vi "confirmINIsettings.vi"() -> ()   [LabVIEW 2012]
doc: "SciScan 1.2 160622"
uses:
  <vilib>/Utility/config.llb/Read Key (String).vi
  GFG/GFGpathGet.vi
  <vilib>/Utility/config.llb/Write Key (Boolean).vi
  <vilib>/Utility/config.llb/Read Key (Boolean).vi
  <vilib>/Utility/config.llb/Write Key (String).vi
  GFG/GFG library.lvlib
  <vilib>/Utility/config.llb/NI_LVConfig.lvlib
panel:
  in  "Fresh config or upgrade?":enum32{"Fresh", "Upgrade"}(radio) caption="1) Start a complete new configuration?"
  in  "PhotoStim Shutter Port":tag="PXI1Slot4/port0/line0" caption="4) Specify the shutter port for the photo stimulation light path"
  in  "DAQ Package":T1(ring) caption="2) Select a DAQ package"
  out "Written files":path[](array[path])
  in  "Load INI variables":bool caption="5) Select optional modules and confirm hardware"
  out "Reso settings complete?":bool
  out "Galvo settings complete?":bool
  out "Loaded scanner configuration":string
  in  "Select modules and confirm hardware":bool caption="6) Select modules and confirm hardware"
  out "Previous INI file settings":path caption="Previous SciScan root path (optional)"
  out "INI to write at....":path
  in  "EXIT":bool
  in  "Switch (Linkbone) Serial Port":refnum<visa-resource-name>=" " caption="3) Specify the detector switch COM port (Linkbone)"
  # "R - Resonant scan mirror   G - Galvo scan mirror"
  # "SciScan Configuration Tool"
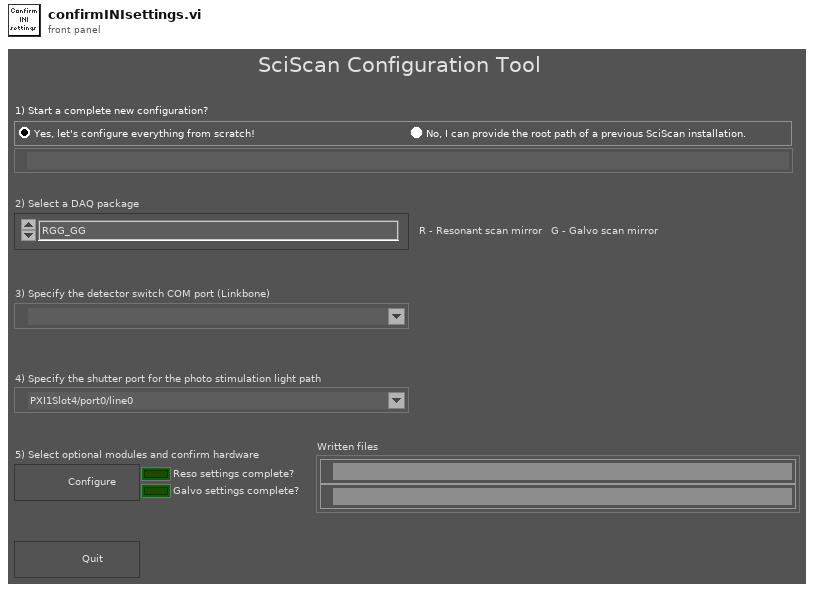
[diagram p1: front panel]
types:
  T1 = enum16{"RGG_GG", "RG_GG", "GG_GG", "RGG", "RG (standalone)", "GG (standalone)"}
  T2 = enum32{"invalid OS target", "Mac OS", "Windows 3.1", "Windows 95/NT", "Solaris 1", "Solaris 2", "HP-UX", "PowerMAX", "Linux", "Irix", "Rhapsody", "BeOS", "AIX", "OSF1", "VxWorks", "PharLap", "Carbon", "RTX", "Windows x64", "Linux x64"}
  T3 = enum8{"Enabled", "Disabled", "Disabled and Grayed Out"}
  T4 = typedef "NI_LVConfig.lvlib/Config Data RefNum.ctl" = refnum<k1>
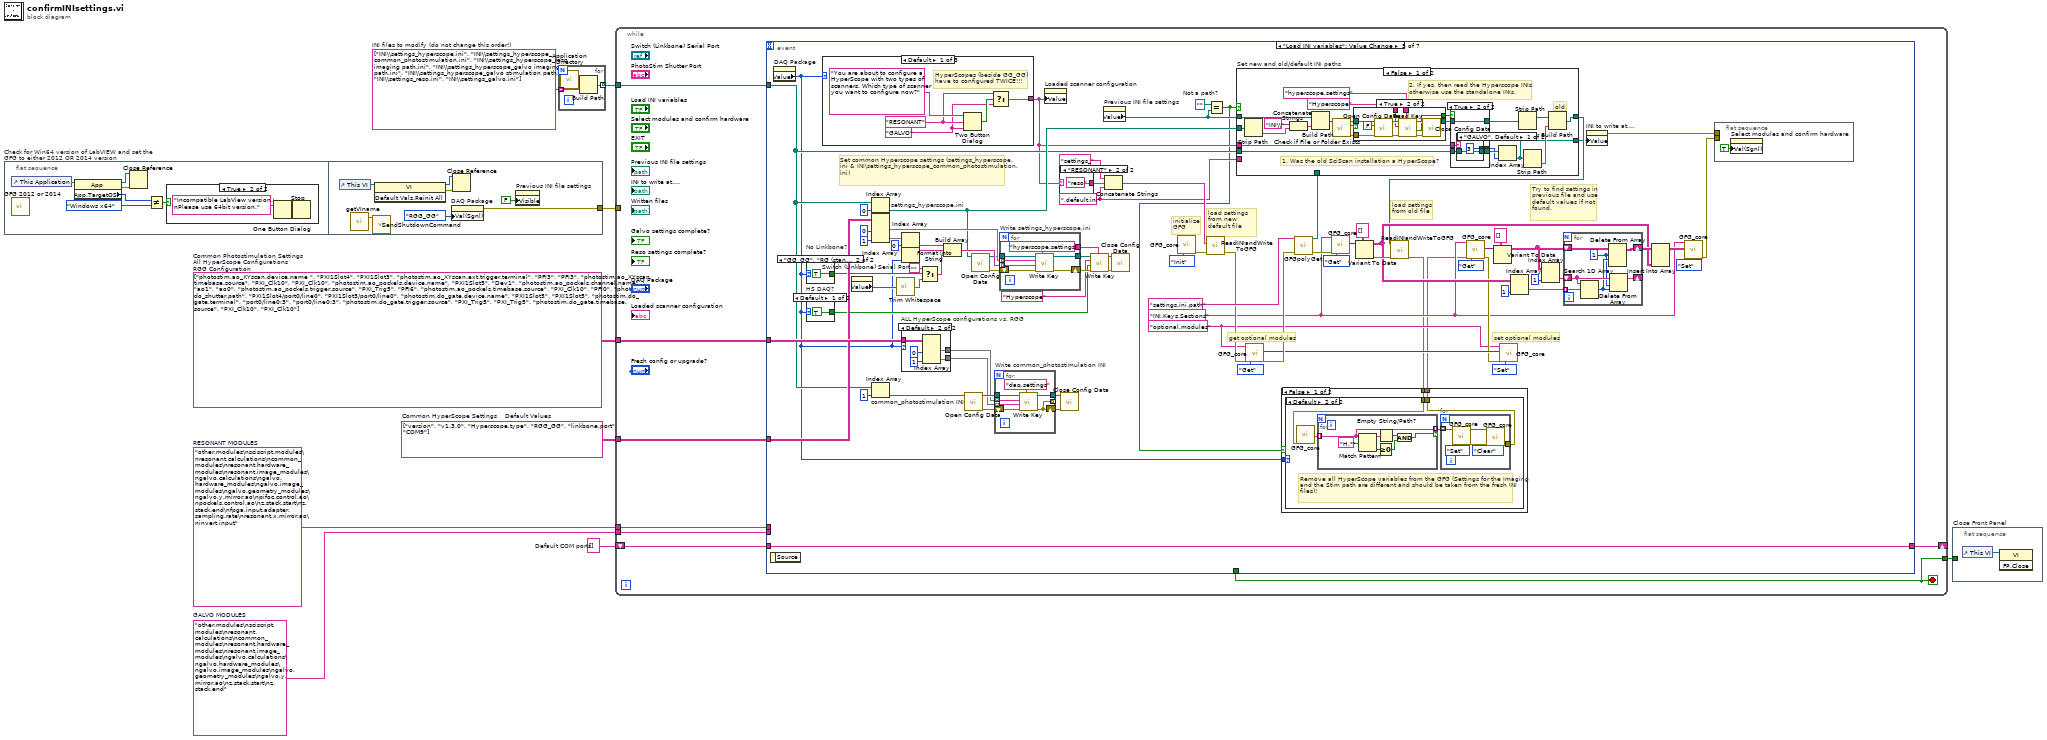
[diagram p0: block diagram]
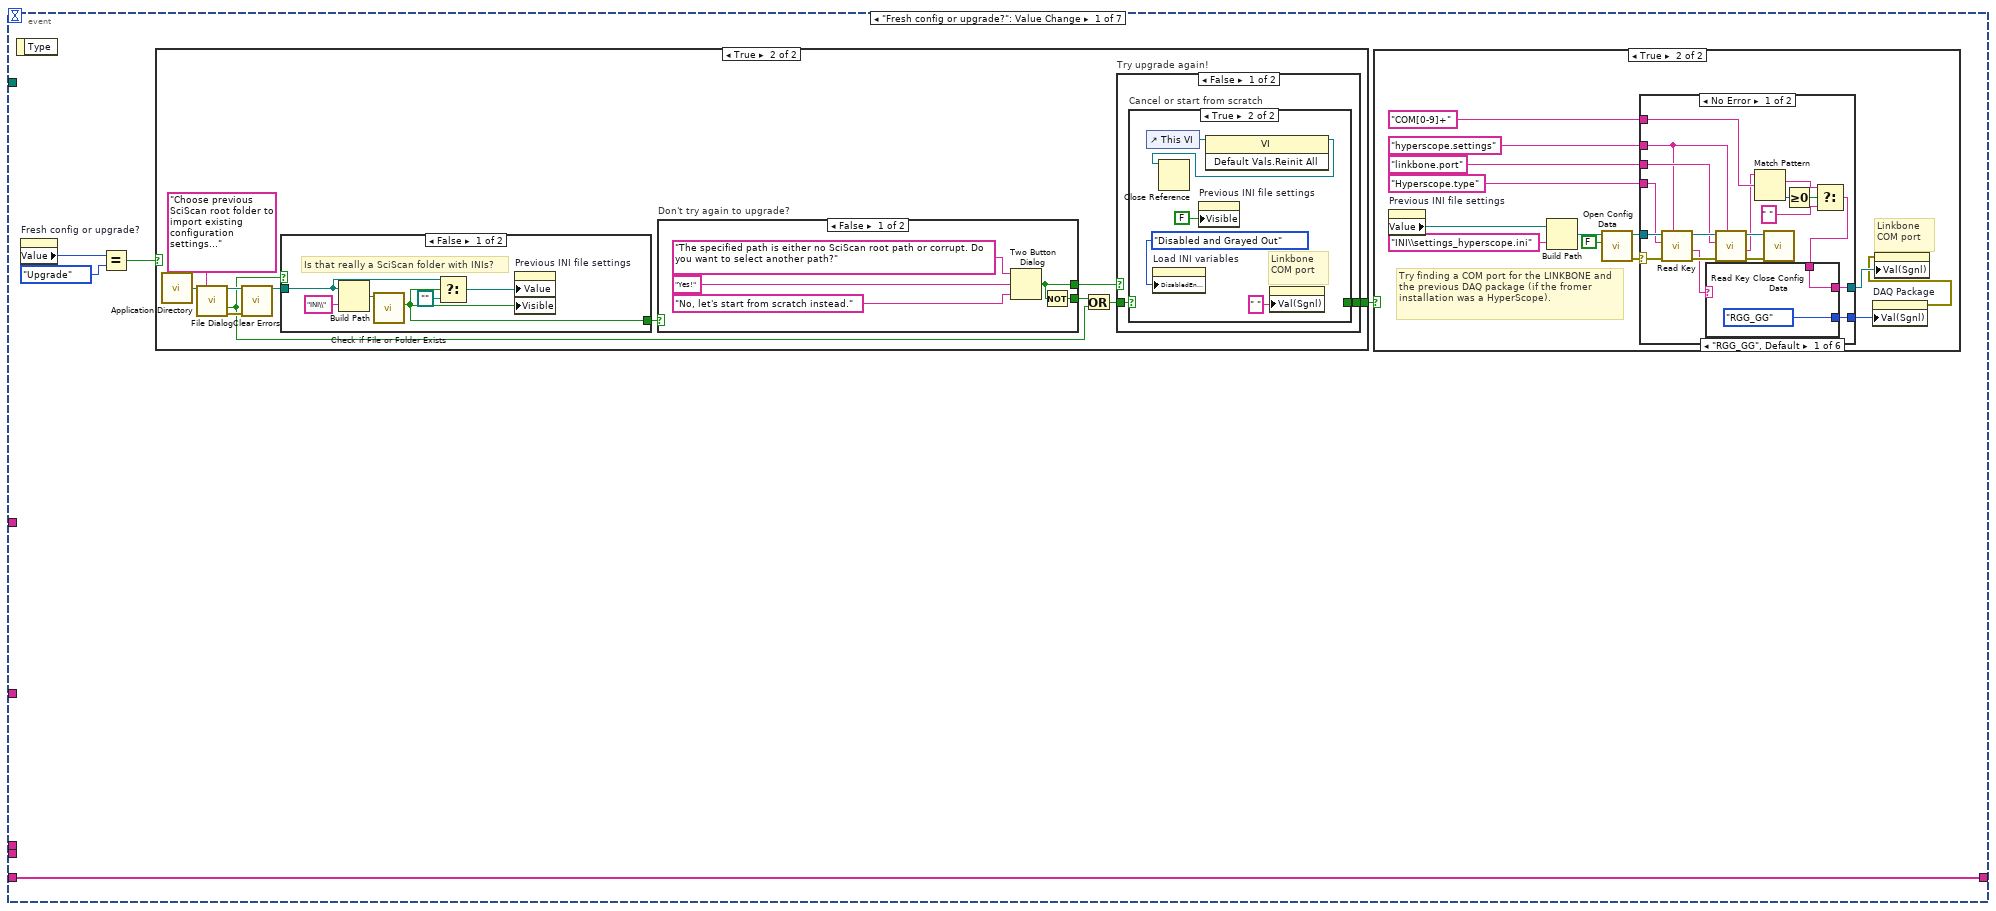
[diagram p3: hidden frame]
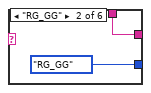
[diagram p5: hidden frame]
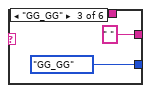
[diagram p6: hidden frame]
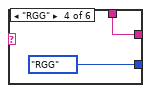
[diagram p7: hidden frame]
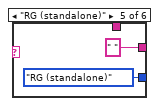
[diagram p8: hidden frame]
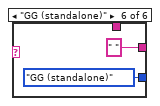
[diagram p9: hidden frame]
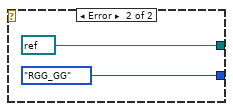
[diagram p10: hidden frame]
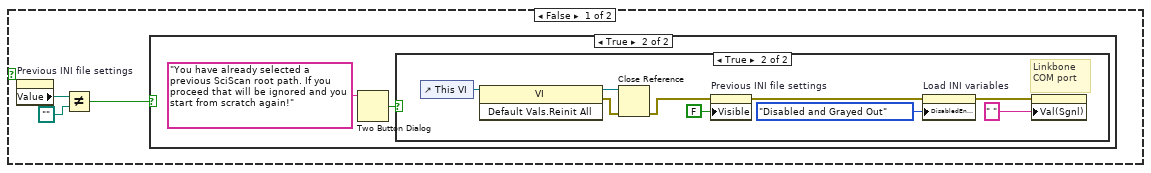
[diagram p11: hidden frame]
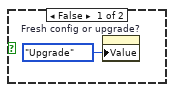
[diagram p13: hidden frame]
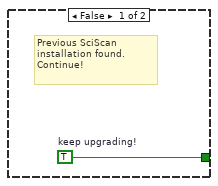
[diagram p15: hidden frame]
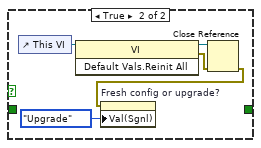
[diagram p16: hidden frame]
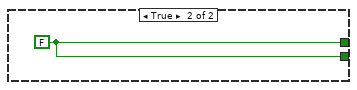
[diagram p17: hidden frame]
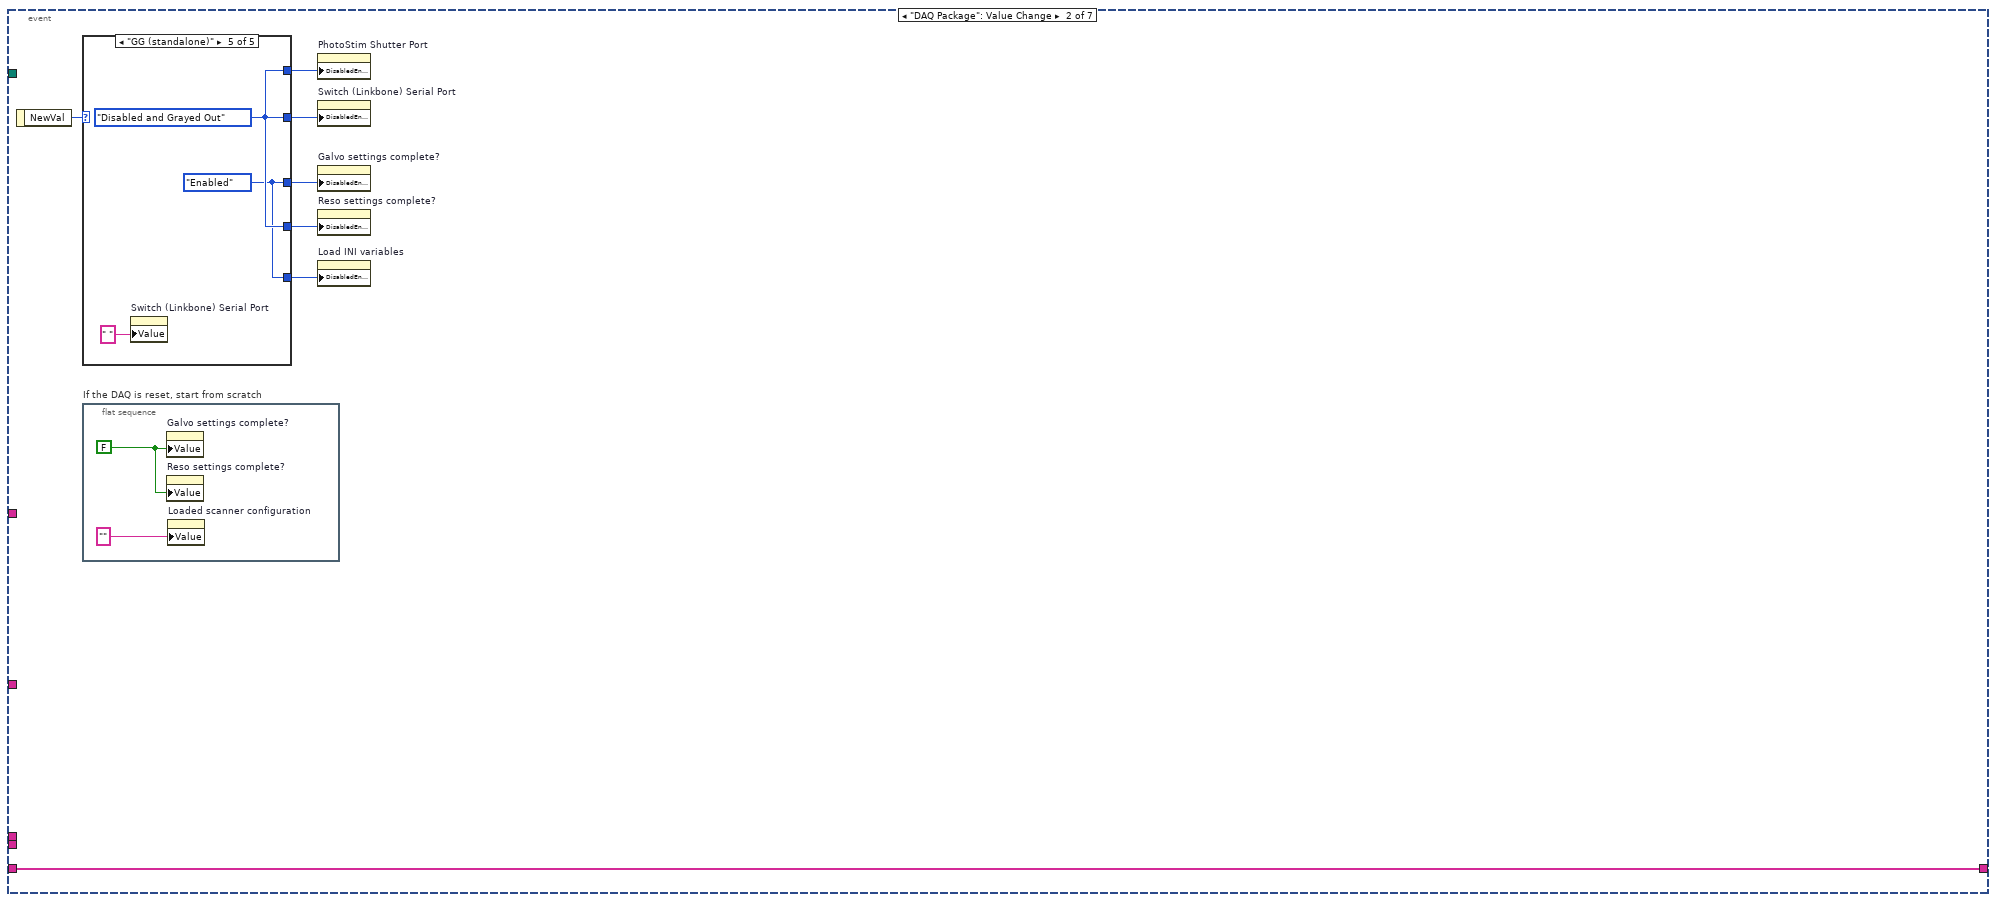
[diagram p18: hidden frame]
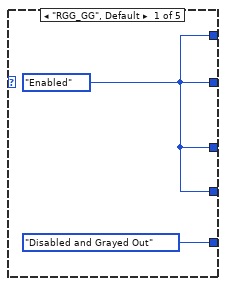
[diagram p19: hidden frame]
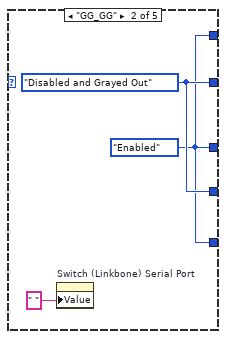
[diagram p20: hidden frame]
diagram:
  w1 = string[] []  # Default COM ports
  w2 = "other.modules\nsciscript.modules\nresonant.calculations\ncommon_modules\nresonant.hardware_modules\nresonant.image_modules\ngalvo.calculations\ngalvo.hardware_modules\ngalvo.image_modules\ngalvo.geometry_modules\ngalvo.y.mirror.ao\npifoc.control.ao\npockels.control.ao\nz.stack.start\nz.stack.end\nfpga.input.adapter.sampling.rate\nresonant.x.mirror.ao\ninvert.input"  # RESONANT MODULES
  w3 = "other.modules\nsciscript.modules\nresonant.calculations\ncommon_modules\nresonant.hardware_modules\nresonant.image_modules\ngalvo.calculations\ngalvo.hardware_modules\ngalvo.image_modules\ngalvo.geometry_modules\ngalvo.y.mirror.ao\nz.stack.start\nz.stack.end"  # GALVO MODULES
  w4 = string[][] [["version", "v1.3.0"], ["Hyperscope.type", "RGG_GG"], ["linkbone.port", "COM9"]]  # Common HyperScope Settings    Default Values
  w7 = string[] ["INI\\settings_hyperscope.ini", "INI\\settings_hyperscope_common_photostimulation.ini", "INI\\settings_hyperscope_reso imaging path.ini", "INI\\settings_hyperscope_galvo imaging path.ini", "INI\\settings_hyperscope_galvo stimulation path.ini", "INI\\settings_reso.ini", "INI\\settings_galvo.ini"]  # INI files to modify (do not change this order!)
  w5 = string[][] [["photostim.ao_XYscan.device.name ", "PXI1Slot4", "PXI1Slot3"], ["photostim.ao_XYscan.ext.trigger.terminal", "PFI3", "PFI3"], ["photostim.ao_XYscan.timebase.source", "PXI_Clk10", "PXI_Clk10"], ["photostim.ao_pockels.device.name", "PXI1Slot5", "Dev1"], ["photostim.ao_pockels.channel.name", "ao1", "ao0"], ["photostim.ao_pockels.trigger.source", "PXI_Trig5", "PFI6"], ["photostim.ao_pockels.timebase.source", "PXI_Clk10", "PFI0"], ["photostim.do_shutter.path", "PXI1Slot4/port0/line0", "PXI1Slot3/port0/line0"], ["photostim.do_gate.device.name", "PXI1Slot5", "PXI1Slot5"], ["photostim.do_gate.terminal", "port0/line0:3", "port0/line0:3"], ["photostim.do_gate.trigger.source", "PXI_Trig5", "PXI_Trig5"], ["photostim.do_gate.timebase.source", "PXI_Clk10", "PXI_Clk10"]]  # Common Photostimulation Settings                 All HyperScope Configurations                       RGG Configuration
  n1 = flat-sequence "Check for Win64 version of LabVIEW and set the GFG to either 2012 OR 2014 version" {
    tunnel: [w20] -> w8
    frame #0 {
      n2 = control-ref of="This Application"() -> (w10:refnum<vi>)
      n3 = call "GFG 2012 or 2014.vi"() -> ()  [unwired: 12 in]
      n4 = property class="App"(reference=w10) -> (reference out=w14:refnum<vi>, error out=w15:errorcluster, "App.TargetOS"=w11:T2)  [unwired: 1 in]
      n5 = Close Reference(reference=w14, error in (no error)=w15) -> ()  [unwired: 1 out]
      n6 = Not Equal?(x=w11, y=T2."Windows x64" ("Application:Target:Operating System")) -> (x != y?=w13:bool)
      n7 = case shown="True" w13 {
        frame False {
        }
        frame True {
          n8 = One Button Dialog(message="Incompatible LabView version.\nPlease use 64bit version." ("source")) -> (true=w16:bool)  [unwired: 1 in]
          n9 = Stop(stop? (T)=w16) -> ()
        }
      }
    }
    frame #1 {
      n10 = control-ref of="This VI"() -> (w22:refnum<vi>)
      n11 = call "getVIname.vi"() -> ("VI name"=w24:string)  [unwired: 19 in]
      n12 = call "SendShutdownCommand.vi"("Source VI"=w24) -> ()  [unwired: 11 in]
      n13 = invoke class="VI" method="Default Vals.Reinit All"(reference=w22) -> (reference out=w19:refnum<vi>, error out=w18:errorcluster)  [unwired: 2 in, 1 out]
      n14 = property on="DAQ Package" class="Enum (strict)"("Val(Sgnl)"=enum16{"RGG_GG", "RG_GG", "GG_GG", "RGG"}."RGG_GG" ("DAQ Package")) -> (error out=w20:errorcluster)  [unwired: 2 in, 1 out]
      n15 = Close Reference(reference=w19, error in (no error)=w18) -> ()  [unwired: 1 out]
      n16 = property on="Previous INI file settings" class="Path"("Visible"=FALSE) -> ()  [unwired: 2 in, 2 out]
    }
  }
  n17 = for {
    tunnel: w7 -> [w26] mode=indexing
    tunnel: [w25] -> w6 mode=indexing
    n18 = call <vilib>:"Application Directory.vi"() -> ("Application Directory"=w27:path)
    n19 = Build Path(base path=w27, name or relative path=w26) -> (appended path=w25:path)
  }
  n20 = while {
    tunnel: [w35] -> w9
    tunnel: w5 -> [w34]
    tunnel: w8 -> [_]
    tunnel: w6 -> [w33]
    tunnel: w4 -> [w32]
    tunnel: w3 -> [w31]
    tunnel: w2 -> [w30]
    shift-right: [w28] -> _
    shift-left: w1 -> [w29]
    stop <- w35 stop-if-true
    n21 = event shown="[4] \"Load INI variables\": Value Change" {
      selector: _ -> [_ _ _ _ _ _ _]
      dyn-events: _ -> [_ _ _ _ _ _ _]
      timeout: _ -> [_ _ _ _ _ _ _]
      tunnel: [_ _ _ _ _ _ w528] -> w35
      tunnel: w34 -> [_ _ _ _ w251 _ _]
      tunnel: w33 -> [_ _ _ _ w186 w393 _]
      tunnel: w32 -> [_ _ _ _ w250 _ _]
      tunnel: w31 -> [_ _ _ _ _ w396 _]
      tunnel: w30 -> [_ _ _ _ _ w395 _]
      tunnel: w29 -> [w40 w139 w166 w169 w248 w381 w527]
      tunnel: [w40 w139 w166 w169 w248 w380 w527] -> w28
      event "Fresh config or upgrade?": Value Change {
        n22 = event-data() -> ()  [unwired: 1 in, 1 out]
        n23 = property on="Fresh config or upgrade?" class="RadioBtnsControl (strict)"() -> ("Value"=w39:enum32{"Fresh", "Upgrade"})  [unwired: 2 in, 2 out]
        n24 = Equal?(x=w39, y=enum32{"Fresh", "Upgrade"}."Upgrade") -> (x = y?=w37:bool)
        n25 = case shown="True" w37 {
          tunnel: [_ w102] -> w36
          frame False {
            n26 = property on="Previous INI file settings" class="Path"() -> ("Value"=w89:path)  [unwired: 2 in, 2 out]
            n27 = Not Equal?(x=w89, y=path "") -> (x != y?=w87:bool)
            n28 = case shown="True" w87 {
              frame False {
              }
              frame True {
                n29 = Two Button Dialog(message="You have already selected a previous SciScan root path. If you proceed that will be ignored and you start from scratch again!") -> (T button?=w90:bool)  [unwired: 2 in]
                n30 = case shown="True" w90 {
                  frame False {
                    n31 = property on="Fresh config or upgrade?" class="RadioBtnsControl (strict)"("Value"=enum32{"Fresh", "Upgrade"}."Upgrade" ("Fresh config or upgrade?")) -> ()  [unwired: 2 in, 2 out]
                  }
                  frame True {
                    # "Linkbone\nCOM port"
                    n32 = control-ref of="This VI"() -> (w101:refnum<vi>)
                    n33 = invoke class="VI" method="Default Vals.Reinit All"(reference=w101) -> (reference out=w97:refnum<vi>, error out=w96:errorcluster)  [unwired: 2 in, 1 out]
                    n34 = Close Reference(reference=w97, error in (no error)=w96) -> (error out=w94:errorcluster)
                    n35 = property on="Previous INI file settings" class="Path"(error in=w94, "Visible"=FALSE) -> (error out=w98:errorcluster)  [unwired: 1 in, 1 out]
                    n36 = property on="Load INI variables" class="Bool"(error in=w98, "DisabledEnum"=T3."Disabled and Grayed Out" ("Disabled")) -> (error out=w95:errorcluster)  [unwired: 1 in, 1 out]
                    n37 = property on="Switch (Linkbone) Serial Port" class="VISAName"(error in=w95, "Val(Sgnl)"=" ") -> ()  [unwired: 1 in, 2 out]
                  }
                }
              }
            }
          }
          frame True {
            n38 = call <vilib>:"Application Directory.vi"() -> ("Application Directory"=w111:path)
            n39 = call "File Dialog"("start path"=w111, "prompt"="Choose previous SciScan root folder to import existing configuration settings...") -> ("selected path"=w109:path, "cancelled"=w106:bool, "error out"=w107:errorcluster)  [unwired: 10 in, 1 out]
            n40 = call <vilib>:"Clear Errors.vi"("error in (no error)"=w107) -> ()  [unwired: 6 in, 1 out]
            n41 = case shown="False" w106 {
              selector: w106 -> [_ w118]
              tunnel: w109 -> [w117 _]
              tunnel: [w112 w118] -> w108
              frame False {
                # "Is that really a SciScan folder with INIs?"
                n42 = Build Path(base path=w117, name or relative path="INI\\") -> (appended path=w115:path)
                n43 = call <vilib>:"Check if File or Folder Exists.vi"("path"=w115) -> ("file or folder exists?"=w112:bool)  [unwired: 8 in, 2 out]
                n44 = Select(t=w117, s=w112, f=path "") -> (s? t:f=w113:path)
                n45 = property on="Previous INI file settings" class="Path"("Value"=w113, "Visible"=w112) -> ()  [unwired: 2 in, 2 out]
              }
              frame True {
              }
            }
            n46 = case "Don't try again to upgrade?" shown="False" w108 {
              tunnel: [w133 w137] -> w104
              tunnel: [w132 w137] -> w103
              frame False {
                n47 = Two Button Dialog(message="The specified path is either no SciScan root path or corrupt. Do you want to select another path?", 1:"No, let's start from scratch instead." ("F button name (\"Cancel\")"), 2:"Yes!" ("T button name (\"OK\")")) -> (T button?=w133:bool)
                n48 = Not(x=w133) -> (.not. x?=w132:bool)
              }
              frame True {
                w137 = FALSE ("T button?")
              }
            }
            n49 = Or(x=w103, y=w106) -> (x .or. y?=w105:bool)
            n50 = case "Try upgrade again!" shown="False" w104 {
              tunnel: w105 -> [w120 _]
              tunnel: [w119 _] -> w102
              frame False {
                n51 = case "Cancel or start from scratch" shown="True" w120 {
                  tunnel: [w121 _] -> w119
                  frame False {
                    w121 = TRUE  # keep upgrading!
                    # "Previous SciScan installation found. Continue!"
                  }
                  frame True {
                    # "Linkbone\nCOM port"
                    n52 = control-ref of="This VI"() -> (w126:refnum<vi>)
                    n53 = property on="Load INI variables" class="Bool"("DisabledEnum"=T3."Disabled and Grayed Out" ("Disabled")) -> ()  [unwired: 2 in, 2 out]
                    n54 = property on="Previous INI file settings" class="Path"("Visible"=FALSE) -> ()  [unwired: 2 in, 2 out]
                    n55 = invoke class="VI" method="Default Vals.Reinit All"(reference=w126) -> (reference out=w125:refnum<vi>)  [unwired: 2 in, 2 out]
                    n56 = Close Reference(reference=w125) -> ()  [unwired: 1 in, 1 out]
                    n57 = property on="Switch (Linkbone) Serial Port" class="VISAName"("Val(Sgnl)"=" ") -> ()  [unwired: 2 in, 2 out]
                  }
                }
              }
              frame True {
                n58 = control-ref of="This VI"() -> (w130:refnum<vi>)
                n59 = invoke class="VI" method="Default Vals.Reinit All"(reference=w130) -> (reference out=w129:refnum<vi>, error out=w128:errorcluster)  [unwired: 2 in, 1 out]
                n60 = Close Reference(reference=w129, error in (no error)=w128) -> (error out=w127:errorcluster)
                n61 = property on="Fresh config or upgrade?" class="RadioBtnsControl (strict)"(error in=w127, "Val(Sgnl)"=enum32{"Fresh", "Upgrade"}."Upgrade" ("Value (Signaling)")) -> ()  [unwired: 1 in, 2 out]
              }
            }
          }
        }
        n62 = case shown="True" w36 {
          frame False {
          }
          frame True {
            # "Try finding a COM port for the LINKBONE and the previous DAQ package (if the fromer installation was a HyperScope)."
            # "Linkbone\nCOM port"
            n63 = property on="Previous INI file settings" class="Path"() -> ("Value"=w48:path)  [unwired: 2 in, 2 out]
            n64 = Build Path(base path=w48, name or relative path="INI\\settings_hyperscope.ini") -> (appended path=w46:path)
            n65 = call <vilib>:"Open Config Data.vi"("create file if necessary (T)"=FALSE, "configuration file path"=w46) -> ("error out"=w45:errorcluster, "refnum"=w53:T4)  [unwired: 7 in, 1 out]
            n66 = case shown="No Error" w45 {
              selector: w45 -> [w63 _]
              tunnel: w53 -> [w72 _]
              tunnel: "Hyperscope.type" ("section") -> [w67 _]
              tunnel: "linkbone.port" ("section") -> [w66 _]
              tunnel: "hyperscope.settings" ("section") -> [w65 _]
              tunnel: [w62 T1."RGG_GG" ("DAQ Package")] -> w44
              tunnel: [w55 refnum<visa-resource-name> refnum ("Switch (Linkbone) Serial Port")] -> w43
              tunnel: "COM[0-9]+" ("regular expression") -> [w60 _]
              frame No Error {
                n67 = call-poly <vilib>:"Read Key.vi"("section"=w65, "error in (no error)"=w63, "key"=w67, "refnum"=w72) -> ("error out"=w70:errorcluster, "value"=w64:string, "refnum out"=w71:T4)  [unwired: 4 in, 1 out]
                n68 = call-poly <vilib>:"Read Key.vi"("section"=w65, "error in (no error)"=w70, "key"=w66, "refnum"=w71) -> ("error out"=w68:errorcluster, "value"=w59:string, "refnum out"=w69:T4)  [unwired: 4 in, 1 out]
                n69 = Match Pattern(string=w59, regular expression=w60) -> (match substring=w58:string, offset past match=w61:i32)  [unwired: 1 in, 2 out]
                n70 = call <vilib>:"Close Config Data.vi"("error in (no error)"=w68, "refnum"=w69) -> ()  [unwired: 8 in, 2 out]
                n71 = Greater Or Equal To 0?(x=w61) -> (x >= 0?=w57:bool)
                n72 = Select(t=w58, s=w57, f=" " ("T button name (\"OK\")")) -> (s? t:f=w56:string)
                n73 = case shown="\"RGG_GG\", Default" w64 {
                  tunnel: [T1."RGG_GG" ("DAQ Package") T1."RG_GG" ("DAQ Package") T1."GG_GG" ("DAQ Package") T1."RGG" ("DAQ Package") T1."RG (standalone)" ("DAQ Package") T1."GG (standalone)" ("DAQ Package")] -> w62
                  tunnel: w56 -> [w73 w75 _ w79 _ _]
                  tunnel: [w73 w75 " " w79 " " " "] -> w55
                  frame "RGG_GG", Default {
                  }
                  frame "RG_GG" {
                  }
                  frame "GG_GG" {
                  }
                  frame "RGG" {
                  }
                  frame "RG (standalone)" {
                  }
                  frame "GG (standalone)" {
                  }
                }
              }
              frame Error {
              }
            }
            n74 = property on="DAQ Package" class="Enum (strict)"("Val(Sgnl)"=w44) -> (error out=w41:errorcluster)  [unwired: 2 in, 1 out]
            n75 = property on="Switch (Linkbone) Serial Port" class="VISAName"(error in=w41, "Val(Sgnl)"=w43) -> ()  [unwired: 1 in, 2 out]
          }
        }
      }
      event "DAQ Package": Value Change {
        n76 = event-data() -> ("NewVal"=w144:T1)  [unwired: 1 in]
        n77 = case shown="\"GG (standalone)\"" w144 {
          tunnel: [w148 w151 w153 w156 w159] -> w141
          tunnel: [w148 w151 w153 w155 w159] -> w143
          tunnel: [w148 w150 w153 w156 w158] -> w142
          tunnel: [w148 w150 w152 w156 w159] -> w140
          tunnel: [T3."Disabled and Grayed Out" ("Disabled") w150 w152 w155 w158] -> w138
          frame "RGG_GG", Default {
            w148 = T3."Enabled" ("Disabled")
          }
          frame "GG_GG" {
            w150 = T3."Enabled" ("Disabled")
            w151 = T3."Disabled and Grayed Out" ("Disabled")
            n78 = property on="Switch (Linkbone) Serial Port" class="VISAName"("Value"=" ") -> ()  [unwired: 2 in, 2 out]
          }
          frame "RGG" {
            w153 = T3."Enabled" ("Disabled")
            w152 = T3."Disabled and Grayed Out" ("Disabled")
          }
          frame "RG (standalone)" {
            w155 = T3."Enabled" ("Disabled")
            w156 = T3."Disabled and Grayed Out" ("Disabled")
            n79 = property on="Switch (Linkbone) Serial Port" class="VISAName"("Value"=" ") -> ()  [unwired: 2 in, 2 out]
          }
          frame "GG (standalone)" {
            w158 = T3."Enabled" ("Disabled")
            w159 = T3."Disabled and Grayed Out" ("Disabled")
            n80 = property on="Switch (Linkbone) Serial Port" class="VISAName"("Value"=" ") -> ()  [unwired: 2 in, 2 out]
          }
        }
        n81 = flat-sequence "If the DAQ is reset, start from scratch" {
          frame #0 {
            w146 = FALSE
            n82 = property on="Galvo settings complete?" class="Bool (strict)"("Value"=w146) -> ()  [unwired: 2 in, 2 out]
            n83 = property on="Reso settings complete?" class="Bool (strict)"("Value"=w146) -> ()  [unwired: 2 in, 2 out]
            n84 = property on="Loaded scanner configuration" class="Str"("Value"="" ("Loaded scanner configuration")) -> ()  [unwired: 2 in, 2 out]
          }
        }
        n85 = property on="PhotoStim Shutter Port" class="DAQmxName"("DisabledEnum"=w140) -> ()  [unwired: 2 in, 2 out]
        n86 = property on="Switch (Linkbone) Serial Port" class="VISAName"("DisabledEnum"=w141) -> ()  [unwired: 2 in, 2 out]
        n87 = property on="Galvo settings complete?" class="Bool (strict)"("DisabledEnum"=w142) -> ()  [unwired: 2 in, 2 out]
        n88 = property on="Reso settings complete?" class="Bool (strict)"("DisabledEnum"=w143) -> ()  [unwired: 2 in, 2 out]
        n89 = property on="Load INI variables" class="Bool"("DisabledEnum"=w138) -> ()  [unwired: 2 in, 2 out]
      }
      event "Switch (Linkbone) Serial Port": Value Change {
        w161 = " "  # VISA control does not change it's display when "" is written back! Use at least " "
        n90 = event-data() -> ("NewVal"=w162:refnum<visa-resource-name>)  [unwired: 1 in]
        n91 = Not Equal?(x=w162, y=w161) -> (x != y?=w160:bool)
        n92 = Select(t=T3."Enabled" ("Disabled"), s=w160, f=T3."Disabled and Grayed Out" ("Disabled")) -> (s? t:f=w163:T3)
        n93 = property on="Load INI variables" class="Bool"("DisabledEnum"=w163) -> ()  [unwired: 2 in, 2 out]
      }
      event "PhotoStim Shutter Port": Value Change {
        n94 = event-data() -> ()  [unwired: 1 in, 1 out]
        n95 = Two Button Dialog(message="Are you sure you want to change the photo stimulation shutter port? The default port is already set correctly for a standard dual path HyperScope.", 1:"Use the default value." ("F button name (\"Cancel\")"), 2:"Apply changes!" ("T button name (\"OK\")")) -> (T button?=w170:bool)
        n96 = case shown="False" w170 {
          frame False {
            n97 = invoke on="PhotoStim Shutter Port" class="DAQmxName" method="Reinit To Default"() -> ()  [unwired: 3 in, 3 out]
          }
          frame True {
          }
        }
      }
      event "Load INI variables": Value Change {
        w177 = ".default.ini" ("name or relative path")
        w221 = "optional.modules" ("Variable Name in")
        w222 = "INI.Keys.Sections" ("Variable Name in")
        # "Try to find settings in previous file and use default values if not found."
        # "load settings from old file"
        # "Set common Hyperscope settings (settings_hyperscope.ini & INI\\settings_hyperscope_common_photostimulation.ini)"
        # "set optional modules"
        # "load settings from new default file"
        # "get optional modules"
        # "initialize GFG"
        n98 = event-data() -> ()  [unwired: 1 in, 1 out]
        n99 = property on="DAQ Package" class="Enum (strict)"() -> ("Value"=w173:T1)  [unwired: 2 in, 2 out]
        n100 = case "No Linkbone?" shown="\"GG_GG\", \"RG (standalone)\", \"GG (standalone)\"" w173 {
          tunnel: [FALSE TRUE] -> w195
          frame Default {
          }
          frame "GG_GG", "RG (standalone)", "GG (standalone)" {
          }
        }
        n101 = case "HS DAQ?" shown="Default" w173 {
          tunnel: [TRUE FALSE] -> w188
          frame Default {
          }
          frame "RG (standalone)", "GG (standalone)" {
          }
        }
        n102 = case shown="Default" w173 {
          tunnel: [w371 "GALVO" ("F button name (\"Cancel\")") "RESONANT" ("T button name (\"OK\")")] -> w181
          frame Default {
            w372 = "GALVO" ("F button name (\"Cancel\")")
            w373 = "RESONANT" ("T button name (\"OK\")")
            # "HyperScopes (beside GG_GG) have to configured TWICE!!!"
            n103 = Two Button Dialog(message="You are about to configure a HyperScope with two types of scanners. Which type of scanner you want to configure now?", 1:w372, 2:w373) -> (T button?=w374:bool)
            n104 = Select(t=w373, s=w374, f=w372) -> (s? t:f=w371:string)
          }
          frame "GG_GG", "GG (standalone)" {
          }
          frame "RG (standalone)" {
          }
        }
        n105 = property on="Switch (Linkbone) Serial Port" class="VISAName"() -> ("Value"=w197:refnum<visa-resource-name>)  [unwired: 2 in, 2 out]
        n106 = Index Array "settings_hyperscope.ini"(array=w186, index=0) -> (element=w187:path)
        n107 = Index Array(array=w250, index (col) #1=0 ("disabled index (col)"), index (col) #2=1 ("index (col)")) -> (element #1=w203:string[], element #2=w207:string[])  [unwired: 2 in]
        n108 = Index Array "common_photostimulation INI"(array=w186, index=1) -> (element=w211:path)
        n109 = call <vilib>:"Trim Whitespace.vi"("string"=w197) -> ("trimmed string"=w196:string)  [unwired: 1 in]
        n110 = Index Array ("VERSION")(array=w207, index=0) -> (element=w205:string)
        n111 = Format Into String(w173) -> (resulting string=w204:string)  [unwired: 3 in, 1 out]
        n112 = case "ALL HyperScope configurations vs. RGG" shown="Default" w173 {
          tunnel: w251 -> [w358 w363]
          tunnel: [w355 w360] -> w215
          tunnel: [w354 w359] -> w216
          frame "RGG" {
            n113 = Index Array(array=w358, index (col) #1=0 ("disabled index (col)"), index (col) #2=2 ("index (col)")) -> (element #1=w354:string[], element #2=w355:string[])  [unwired: 2 in]
          }
          frame Default {
            n114 = Index Array(array=w363, index (col) #1=0 ("disabled index (col)"), index (col) #2=1 ("index (col)")) -> (element #1=w359:string[], element #2=w360:string[])  [unwired: 2 in]
          }
        }
        n115 = Select(t="", s=w195, f=w196) -> (s? t:f=w200:string)
        n116 = Build Array(w205, w204, w200) -> (w202:string[])
        n117 = call <vilib>:"Open Config Data.vi"("configuration file path"=w211) -> ("error out"=w217:errorcluster, "refnum"=w218:T4)  [unwired: 8 in, 1 out]
        n118 = call <vilib>:"Open Config Data.vi"("configuration file path"=w187) -> ("error out"=w198:errorcluster, "refnum"=w199:T4)  [unwired: 8 in, 1 out]
        n119 = for "Write common_photostimulation INI" {
          tunnel: w218 -> [w352]
          tunnel: w216 -> [w350] mode=indexing
          tunnel: w215 -> [w347] mode=indexing
          shift-right: [w348] -> w213
          shift-left: w217 -> [w351]
          tunnel: [w349] -> w214
          tunnel: [w348] -> _ mode=indexing
          n120 = call-poly <vilib>:"Write Key.vi"("section"="daq.settings", "error in (no error)"=w351, "value"=w347, "key"=w350, "refnum"=w352) -> ("error out"=w348:errorcluster, "refnum out"=w349:T4)  [unwired: 4 in, 1 out]
        }
        n121 = for "Write settings_hyperscope.ini" {
          tunnel: w199 -> [w346]
          tunnel: [w343] -> w193
          shift-right: [w344] -> w194
          shift-left: w198 -> [w345]
          tunnel: w203 -> [w341] mode=indexing
          tunnel: w202 -> [w342] mode=indexing
          tunnel: [w340] -> w192
          w340 = "hyperscope.settings" ("section")
          n122 = call-poly <vilib>:"Write Key.vi"("section"=w340, "error in (no error)"=w345, "value"=w342, "key"=w341, "refnum"=w346) -> ("error out"=w344:errorcluster, "refnum out"=w343:T4)  [unwired: 4 in, 1 out]
        }
        n123 = property on="Loaded scanner configuration" class="Str"("Value"=w181) -> ()  [unwired: 2 in, 2 out]
        n124 = case shown="\"RESONANT\"" w181 {
          tunnel: ["galvo" ("name or relative path") "reso" ("name or relative path")] -> w179
          frame "GALVO", Default {
          }
          frame "RESONANT" {
          }
        }
        n125 = call <vilib>:"Close Config Data.vi"("error in (no error)"=w213, "refnum"=w214) -> ()  [unwired: 8 in, 2 out]
        n126 = call-poly <vilib>:"Write Key.vi"("section"=w192, "error in (no error)"=w194, "value"=w188, "key"="Hyperscope" ("section"), "refnum"=w193) -> ("error out"=w191:errorcluster, "refnum out"=w190:T4)  [unwired: 4 in, 1 out]
        n127 = property on="Previous INI file settings" class="Path"() -> ("Value"=w183:path)  [unwired: 2 in, 2 out]
        n128 = Concatenate Strings("settings_" ("name or relative path"), w179, w177) -> (w178:string)
        n129 = call <vilib>:"Close Config Data.vi"("error in (no error)"=w191, "refnum"=w190) -> ()  [unwired: 8 in, 2 out]
        n130 = call "GFG_core.vi"("Action"=enum16{"Init", "Set", "Get"}."Init") -> ("error out"=w246:errorcluster)  [unwired: 12 in, 6 out]
        n131 = call "ReadINIandWriteToGFG.vi"("error in (no error)"=w246, "name or relative path"=w178) -> ("error out"=w227:errorcluster)  [unwired: 9 in]
        n132 = Equal? "Not a path?"(x=path "", y=w183) -> (x = y?=w172:bool)
        n133 = call "GFG_core.vi"("Variable Name in"=w221, "error in (no error)"=w227, "Action"=enum16{"Init", "Set", "Get", "Clear"}."Get") -> ("Variant Out"=w225:variant, "error out"=w226:errorcluster)  [unwired: 10 in, 5 out]
        n134 = call-poly "GFGpolyGet.vi"("error in (no error)"=w226, "Variable Name in"="settings.ini.path") -> ("error out"=w240:errorcluster, "Path"=w185:path)  [unwired: 7 in, 1 out]
        n135 = case "Set new and old/default INI paths" shown="False" w172 {
          tunnel: w183 -> [w296 _]
          tunnel: w187 -> [w297 _]
          tunnel: w181 -> [w288 _]
          tunnel: w186 -> [w287 _]
          tunnel: [w280 w335] -> w184
          tunnel: w185 -> [_ w335]
          tunnel: [w279 w330] -> w176
          tunnel: w177 -> [_ w331]
          frame False {
            # "old"
            # "2. If yes, then read the Hyperscope INIs, otherwise use the standalone INIs."
            # "1. Was the old SciScan installation a HyperScope?"
            n136 = Strip Path(path=w297) -> (name=w276:string)  [unwired: 1 out]
            n137 = Concatenate Strings("INI\\" ("string"), w276) -> (w278:string)
            n138 = Build Path(base path=w296, name or relative path=w278) -> (appended path=w295:path)
            n139 = call <vilib>:"Check if File or Folder Exists.vi"("path"=w295) -> ("error out"=w293:errorcluster, "file or folder exists?"=w290:bool, "dup path"=w294:path)  [unwired: 8 in]
            n140 = case shown="True" w290 {
              tunnel: w294 -> [w316 w328]
              tunnel: w293 -> [_ w327]
              tunnel: "Hyperscope" ("section") -> [_ w323]
              tunnel: "hyperscope.settings" ("section") -> [_ w322]
              tunnel: [FALSE ("value") w319] -> w289
              tunnel: [w316 w318] -> w284
              frame False {
              }
              frame True {
                n141 = call <vilib>:"Open Config Data.vi"("error in (no error)"=w327, "create file if necessary (T)"=FALSE, "configuration file path"=w328) -> ("error out"=w324:errorcluster, "refnum"=w325:T4)  [unwired: 6 in, 1 out]
                n142 = call-poly <vilib>:"Read Key.vi"("section"=w322, "error in (no error)"=w324, "key"=w323, "refnum"=w325) -> ("error out"=w320:errorcluster, "value"=w319:bool, "refnum out"=w321:T4)  [unwired: 4 in, 1 out]
                n143 = call <vilib>:"Close Config Data.vi"("error in (no error)"=w320, "refnum"=w321) -> ("file path"=w318:path)  [unwired: 8 in, 1 out]
              }
            }
            n144 = case shown="True" w289 {
              tunnel: w288 -> [w302 w311]
              tunnel: w287 -> [w300 w310]
              tunnel: [w301 w309] -> w285
              tunnel: [w299 w308] -> w286
              tunnel: w284 -> [w298 w307]
              tunnel: [w298 w307] -> w283
              frame False {
                n145 = case shown="\"RESONANT\"" w302 {
                  tunnel: [6 ("index") 5 ("index")] -> w301
                  tunnel: w300 -> [w303 w305]
                  tunnel: [w303 w305] -> w299
                  frame "GALVO", Default {
                  }
                  frame "RESONANT" {
                  }
                }
              }
              frame True {
                n146 = case shown="\"GALVO\", Default" w311 {
                  tunnel: [3 ("index") 2 ("index")] -> w309
                  tunnel: w310 -> [w312 w314]
                  tunnel: [w312 w314] -> w308
                  frame "GALVO", Default {
                  }
                  frame "RESONANT" {
                  }
                }
              }
            }
            n147 = Index Array(array=w286, index=w285) -> (element=w279:path)
            n148 = Strip Path(path=w283) -> (stripped path=w282:path)  [unwired: 1 out]
            n149 = Strip Path(path=w279) -> (name=w281:string)  [unwired: 1 out]
            n150 = Build Path(base path=w282, name or relative path=w281) -> (appended path=w280:path)
          }
          frame True {
            # "No previous SciScan installation specified / found."
            n151 = Strip Path(path=w335) -> (stripped path=w334:path, name=w333:string)
            n152 = Search and Replace String(input string=w333, search string=w331, replace string=".ini" ("replace string (\"\")")) -> (result string=w332:string)  [unwired: 5 in, 3 out]
            n153 = Build Path(base path=w334, name or relative path=w332) -> (appended path=w330:path)
          }
        }
        n154 = call "GFG_core.vi"("Variable Name in"=w222, "error in (no error)"=w240, "Action"=enum16{"Init", "Set", "Get"}."Get") -> ("Variant Out"=w244:variant)  [unwired: 10 in, 6 out]
        n155 = Variant To Data(type=string[][] [], Variant=w244) -> (data=w230:string[][], error out=w242:errorcluster)  [unwired: 1 in]
        n156 = call "ReadINIandWriteToGFG.vi"("error in (no error)"=w242, "configuration file path"=w184) -> ("error out"=w175:errorcluster)  [unwired: 9 in]
        n157 = case shown="False" w172 {
          tunnel: w175 -> [w254 w273]
          tunnel: [w253 w273] -> w174
          tunnel: w173 -> [w252 _]
          frame False {
            n158 = case shown="Default" w252 {
              tunnel: w254 -> [w255 w257]
              tunnel: [w255 w256] -> w253
              frame "GG_GG", "RG (standalone)", "GG (standalone)" {
              }
              frame Default {
                # "Remove all HyperScope variables from the GFG (Settings for the Imaging and the Stim path are different and should be taken from the fresh INI files)!"
                n159 = call "GFG_core.vi"("error in (no error)"=w257) -> ("All Variable Names Out"=w259:string[])  [unwired: 12 in, 6 out]
                n160 = for {
                  tunnel: w259 -> [w261] mode=indexing
                  tunnel: [w261] -> w258 mode=indexing if=w260
                  n161 = Match Pattern(string=w261, regular expression="H.*") -> (before substring=w264:string, offset past match=w265:i32)  [unwired: 1 in, 2 out]
                  n162 = Greater Or Equal To 0?(x=w265) -> (x >= 0?=w262:bool)
                  n163 = Empty String/Path?(string/path=w264) -> (empty?=w263:bool)
                  n164 = And(x=w263, y=w262) -> (x .and. y?=w260:bool)
                }
                n165 = for {
                  tunnel: w258 -> [w272] mode=indexing
                  tunnel: [w267] -> w256
                  n166 = call "GFG_core.vi"("Variable Name in"=w272, "Action"=enum16{"Init", "Set", "Get", "Clear"}."Set") -> ("Variable Name Out"=w270:string, "error out"=w269:errorcluster)  [unwired: 11 in, 5 out]
                  n167 = call "GFG_core.vi"("Variable Name in"=w270, "error in (no error)"=w269, "Action"=enum16{"Init", "Set", "Get", "Clear"}."Clear") -> ("error out"=w267:errorcluster)  [unwired: 10 in, 6 out]
                }
              }
            }
          }
          frame True {
          }
        }
        n168 = call "GFG_core.vi"("Variable Name in"=w222, "error in (no error)"=w174, "Action"=enum16{"Init", "Set", "Get"}."Get") -> ("Variant Out"=w238:variant, "error out"=w223:errorcluster)  [unwired: 10 in, 5 out]
        n169 = Variant To Data(type=string[][] [], Variant=w238) -> (data=w233:string[][])  [unwired: 1 in, 1 out]
        n170 = call "GFG_core.vi"("Variable Name in"=w221, "Variant in"=w225, "error in (no error)"=w223, "Action"=enum16{"Init", "Set", "Get", "Clear"}."Set") -> ()  [unwired: 9 in, 7 out]
        n171 = Index Array(array=w230, index (col)=1 ("disabled index (col)")) -> (element=w235:string[])  [unwired: 1 in]
        n172 = Index Array(array=w233, index (col)=1 ("disabled index (col)")) -> (element=w232:string[])  [unwired: 1 in]
        n173 = for {
          shift-right: [w365] -> w231
          shift-left: w233 -> [w367]
          tunnel: w235 -> [w370] mode=indexing
          shift-right: [w368] -> _
          shift-left: w232 -> [w369]
          w364 = 1 ("length")
          n174 = Search 1D Array(1D array=w369, element=w370) -> (index of element=w366:i32)  [unwired: 1 in]
          n175 = Delete From Array(array=w367, length=w364, index (row)=w366) -> (array with subset deleted=w365:string[][])  [unwired: 1 in, 1 out]
          n176 = Delete From Array(array=w369, length=w364, index=w366) -> (array with subset deleted=w368:string[])  [unwired: 1 out]
        }
        n177 = property on="INI to write at...." class="Path"("Value"=w176) -> (error out=w249:errorcluster)  [unwired: 2 in, 1 out]
        n178 = Insert Into Array(array=w231, new element=w230) -> (w228:string[][])  [unwired: 2 in]
        n179 = call "GFG_core.vi"("Variable Name in"=w222, "Variant in"=w228, "Action"=enum16{"Init", "Set", "Get"}."Set") -> ("error out"=w219:errorcluster)  [unwired: 10 in, 6 out]
        n180 = flat-sequence {
          tunnel: w249 -> [_]
          tunnel: w219 -> [_]
          frame #0 {
            n181 = property on="Select modules and confirm hardware" class="Bool (strict)"("Val(Sgnl)"=TRUE) -> ()  [unwired: 2 in, 2 out]
          }
        }
      }
      event "Select modules and confirm hardware": Value Change {
        w383 = T3."Enabled" ("x")
        n182 = event-data() -> ()  [unwired: 1 in, 1 out]
        n183 = property on="DAQ Package" class="Enum (strict)"() -> ("Value"=w392:T1)  [unwired: 2 in, 2 out]
        n184 = property on="Loaded scanner configuration" class="Str"() -> ("Value"=w394:string)  [unwired: 2 in, 2 out]
        n185 = property on="Select modules and confirm hardware" class="Bool (strict)"("Value"=FALSE) -> ()  [unwired: 2 in, 2 out]
        n186 = case shown="\"GALVO\"" w394 {
          tunnel: w392 -> [_ w426 w467]
          tunnel: w396 -> [_ _ w469]
          tunnel: w395 -> [_ w427 _]
          tunnel: w393 -> [_ w425 w468]
          tunnel: [_ w419 w462] -> w382
          tunnel: w381 -> [w416 w418 w459]
          tunnel: [w416 w417 w458] -> w380
          frame Default {
          }
          frame "RESONANT" {
            # "WRITE SETTINGS TO INI FILE"
            n187 = case shown="\"RG (standalone)\"" w426 {
              tunnel: w425 -> [w436 _]
              tunnel: [w434 w437] -> w422
              frame Default {
                n188 = Index Array(array=w436, index=2) -> (element=w434:path)
              }
              frame "RG (standalone)" {
                n189 = property on="INI to write at...." class="Path"() -> ("Value"=w437:path)  [unwired: 2 in, 2 out]
              }
            }
            n190 = flat-sequence {
              tunnel: w422 -> [w444]
              tunnel: [w444] -> w433
              tunnel: w433 -> [w450]
              tunnel: [w450] -> w432
              tunnel: [w446] -> w431
              tunnel: w432 -> [w454]
              tunnel: [w454] -> w430
              tunnel: w431 -> [w453]
              tunnel: w418 -> [w452]
              tunnel: [w451] -> w417
              tunnel: w430 -> [w457]
              tunnel: w429 -> [w456]
              tunnel: [w455] -> w423
              frame #0 {
                n191 = call "confirm hardware config.vi"() -> ()  [unwired: 12 in]
              }
              frame #1 {
                n192 = call "list all modules.vi"("resonant or galvo? (T is reso)"=TRUE) -> ("inactive modules"=w448:string[], "optional modules"=w447:string[], "required modules"=w449:string[])  [unwired: 8 in]
                n193 = call "confirm modules.vi"("inactive modules IN"=w448, "optional modules IN"=w447, "required modules IN"=w449) -> ("optional modules out"=w446:string[])  [unwired: 6 in, 2 out]
              }
              frame #2 {
                n194 = call "choose com ports.vi"("Default COM ports IN"=w452, "optional modules"=w453) -> ("Default COM ports OUT"=w451:string[])  [unwired: 9 in]
              }
              frame #3 {
                n195 = call "ReadGFGandWriteToINI.vi"("remove keys"=w456, "Path"=w457) -> ("error out"=w455:errorcluster)  [unwired: 9 in]
              }
            }
            n196 = while {
              tunnel: "" -> [w441]
              tunnel: [w439] -> w429 mode=indexing
              tunnel: w427 -> [w438]
              i -> [w442]
              stop <- w440 stop-if-true
              n197 = Pick Line(string ("")=w441, multi-line string=w438, line index=w442) -> (output string=w439:string)
              n198 = String Length(string=w439) -> (length=w443:i32)
              n199 = Equal To 0?(x=w443) -> (x = 0?=w440:bool)
            }
            n200 = property on="Reso settings complete?" class="Bool (strict)"(error in=w423, "Value"=TRUE ("Reso settings complete?")) -> (error out=w421:errorcluster)  [unwired: 1 in, 1 out]
            n201 = Build Array(w422) -> (w420:path[])
            n202 = property on="Written files" class="Arr (strict)"(error in=w421, "Value"=w420) -> (error out=w419:errorcluster)  [unwired: 1 in, 1 out]
          }
          frame "GALVO" {
            # "WRITE SETTINGS TO INI FILE(S)"
            n203 = case shown="\"GG (standalone)\"" w467 {
              tunnel: w468 -> [w481 _]
              tunnel: [w476 w483] -> w463
              tunnel: ["PXI1Slot3/port0/line0" ("Default IMAGING shutter") "Dev1/port0/line0" ("Variable Name in")] -> w461
              frame Default {
                n204 = Index Array(array=w481, index #1=3 ("index"), index #2=4 ("index")) -> (element #1=w478:path, element #2=w477:path)
                n205 = Build Array(w478, w477) -> (w476:path[])
              }
              frame "GG (standalone)" {
                n206 = property on="INI to write at...." class="Path"() -> ("Value"=w484:path)  [unwired: 2 in, 2 out]
                n207 = Build Array(w484) -> (w483:path[])
              }
            }
            n208 = flat-sequence {
              tunnel: [w496] -> w474
              tunnel: [w492] -> w473
              tunnel: w463 -> [w496]
              tunnel: w461 -> [w491]
              tunnel: [w491] -> w460
              tunnel: w474 -> [w501]
              tunnel: [w501] -> w472
              tunnel: w473 -> [w500]
              tunnel: w460 -> [w499]
              tunnel: w459 -> [w498]
              tunnel: [w497] -> w458
              tunnel: w472 -> [w504]
              tunnel: w471 -> [w503]
              tunnel: [w502] -> w466
              frame #0 {
                n209 = call "list all modules.vi"() -> ("inactive modules"=w494:string[], "optional modules"=w493:string[], "required modules"=w495:string[])  [unwired: 9 in]
                n210 = call "confirm modules.vi"("inactive modules IN"=w494, "optional modules IN"=w493, "required modules IN"=w495) -> ("optional modules out"=w492:string[])  [unwired: 6 in, 2 out]
              }
              frame #1 {
                n211 = call "choose com ports.vi"("Default COM ports IN"=w498, "Default IMAGING shutter"=w499, "optional modules"=w500) -> ("Default COM ports OUT"=w497:string[])  [unwired: 8 in]
              }
              frame #2 {
                n212 = for {
                  tunnel: w504 -> [w509] mode=indexing
                  tunnel: [w508] -> w502
                  tunnel: w503 -> [w506]
                  i -> [w507]
                  n213 = Greater Than 0?(x=w507) -> (x > 0?=w505:bool)
                  n214 = case "Write the correct shutter routing for the photostim path (i >0)!!!" shown="True" w505 {
                    tunnel: w509 -> [w512 w515]
                    tunnel: [w511 w516] -> w508
                    tunnel: w506 -> [w510 w517]
                    frame False {
                      n215 = call "ReadGFGandWriteToINI.vi"("remove keys"=w510, "Path"=w512) -> ("error out"=w511:errorcluster)  [unwired: 9 in]
                    }
                    frame True {
                      n216 = flat-sequence {
                        tunnel: w515 -> [w519]
                        tunnel: [w519] -> w513
                        tunnel: [w522] -> w514
                        tunnel: w513 -> [w522]
                        tunnel: w517 -> [w526]
                        tunnel: [w525] -> w516
                        tunnel: w514 -> [w524]
                        frame #0 {
                          n217 = property on="PhotoStim Shutter Port" class="DAQmxName"() -> ("Value"=w518:string)  [unwired: 2 in, 2 out]
                          n218 = call "GFG_core.vi"("Variable Name in"="shutter.DO", "Variant in"=w518, "Action"=enum16{"Init", "Set", "Get", "Clear"}."Set") -> ()  [unwired: 10 in, 7 out]
                        }
                        frame #1 {
                          n219 = Wait (ms)(milliseconds to wait=u32 20) -> ()  [unwired: 1 out]
                        }
                        frame #2 {
                          n220 = call "ReadGFGandWriteToINI.vi"("remove keys"=w526, "Path"=w524) -> ("error out"=w525:errorcluster)  [unwired: 9 in]
                        }
                      }
                    }
                  }
                }
              }
            }
            n221 = while {
              tunnel: "" -> [w488]
              tunnel: [w486] -> w471 mode=indexing
              tunnel: w469 -> [w485]
              i -> [w489]
              stop <- w487 stop-if-true
              n222 = Pick Line(string ("")=w488, multi-line string=w485, line index=w489) -> (output string=w486:string)
              n223 = String Length(string=w486) -> (length=w490:i32)
              n224 = Equal To 0?(x=w490) -> (x = 0?=w487:bool)
            }
            n225 = property on="Galvo settings complete?" class="Bool (strict)"(error in=w466, "Value"=TRUE) -> (error out=w464:errorcluster)  [unwired: 1 in, 1 out]
            n226 = property on="Written files" class="Arr (strict)"(error in=w464, "Value"=w463) -> (error out=w462:errorcluster)  [unwired: 1 in, 1 out]
          }
        }
        n227 = property on="Galvo settings complete?" class="Bool (strict)"(error in=w382) -> ("DisabledEnum"=w385:T3, "Value"=w389:bool)  [unwired: 1 in, 2 out]
        n228 = property on="Reso settings complete?" class="Bool (strict)"(error in=w382) -> ("DisabledEnum"=w384:T3, "Value"=w390:bool)  [unwired: 1 in, 2 out]
        n229 = Equal?(x=w383, y=w385) -> (x = y?=w386:bool)
        n230 = Equal?(x=w383, y=w384) -> (x = y?=w387:bool)
        n231 = And(x=w386, y=w387) -> (x .and. y?=w388:bool)
        n232 = case shown="True" w388 {
          tunnel: w389 -> [w398 w405]
          tunnel: w390 -> [w397 w403]
          tunnel: [w400 w404] -> w391
          frame False {
            n233 = Or(x=w398, y=w397) -> (x .or. y?=w399:bool)
            n234 = case shown="False" w399 {
              tunnel: ["Could not load the settings properly!" ("message") "The configuration has been completed. The configuration tool can be quit now." ("message")] -> w400
              frame False {
              }
              frame True {
              }
            }
          }
          frame True {
            n235 = And(x=w405, y=w403) -> (x .and. y?=w406:bool)
            n236 = case shown="False" w406 {
              tunnel: w405 -> [w409 _]
              tunnel: [w408 "The configuration has been completed for both scanner types. The configuration tool can be quit now." ("message")] -> w404
              tunnel: w403 -> [w407 _]
              frame False {
                n237 = case shown="False" w409 {
                  tunnel: [w410 "The configuration has been completed for the Galvo scanner. Please configure  the Resonant scanner now (again step 5)." ("message")] -> w408
                  tunnel: w407 -> [w411 _]
                  frame False {
                    n238 = case shown="False" w411 {
                      tunnel: ["Could not load the settings properly!" ("message") "The configuration has been completed for the Resonant scanner. Please configure the Galvo scanner now (again step 5)." ("message")] -> w410
                      frame False {
                      }
                      frame True {
                      }
                    }
                  }
                  frame True {
                  }
                }
              }
              frame True {
              }
            }
          }
        }
        n239 = One Button Dialog(message=w391) -> ()  [unwired: 1 in, 1 out]
      }
      event "EXIT": Value Change {
        n240 = event-data() -> ()  [unwired: 1 in, 1 out]
        n241 = property on="Galvo settings complete?" class="Bool (strict)"() -> ("DisabledEnum"=w541:T3, "Value"=w538:bool)  [unwired: 2 in, 2 out]
        n242 = property on="Reso settings complete?" class="Bool (strict)"() -> ("DisabledEnum"=w533:T3, "Value"=w532:bool)  [unwired: 2 in, 2 out]
        n243 = Equal?(x=T3."Enabled", y=w541) -> (x = y?=w539:bool)
        n244 = Equal?(x=T3."Enabled", y=w533) -> (x = y?=w535:bool)
        n245 = Select(t=w538, s=w539, f=TRUE) -> (s? t:f=w531:bool)
        n246 = Select(t=w532, s=w535, f=TRUE) -> (s? t:f=w530:bool)
        n247 = And(x=w531, y=w530) -> (x .and. y?=w529:bool)
        n248 = case shown="False" w529 {
          tunnel: [w542 TRUE] -> w528
          frame False {
            n249 = Two Button Dialog(message="You did not finish the configuration yet.\nAre you sure you want to quit?") -> (T button?=w542:bool)  [unwired: 2 in]
          }
          frame True {
          }
        }
      }
    }
  }
  n250 = flat-sequence "Close Front Panel" {
    tunnel: w9 -> [_]
    frame #0 {
      n251 = control-ref of="This VI"() -> (w545:refnum<vi>)
      n252 = invoke class="VI" method="FP.Close"(reference=w545) -> ()  [unwired: 2 in, 3 out]
    }
  }
